vi "Determine Controller.vi"(7 "Processing In":refnum<class "Processing.lvclass">, 11 "PathRegex Router in":refnum<class "PathRegex Router.lvclass">) -> (0 "error out":errorcluster, 2 "Controller":refnum<class "Controller.lvclass">, 5 "Processing":refnum<class "Processing.lvclass">)   [LabVIEW 2020, in "HTTP Server.lvlib" / "PathRegex Router.lvclass"]
uses:
  PathRegex Router.lvclass
  PathRegex Router.lvclass/PathRegex Router.ctl
  lv-http-util/HTTP Utils/Request/Request.lvclass
  Controller/Controller.lvclass
  Processing/Processing.lvclass
  lv-uri/URI/URI/URI.lvclass
  lv-uri/URI/URI.lvlib
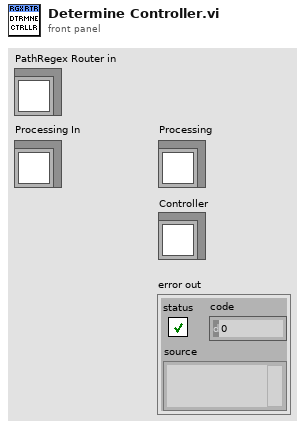
[diagram p1: front panel]
types:
  T1 = typedef "HTTP Server.lvlib/Controller Map.ctl" = map{T2, refnum<class "Controller.lvclass">}
  T2 = typedef "HTTP Server.lvlib/Priority.ctl" = cluster{"Entity":u16, "Index":u16}
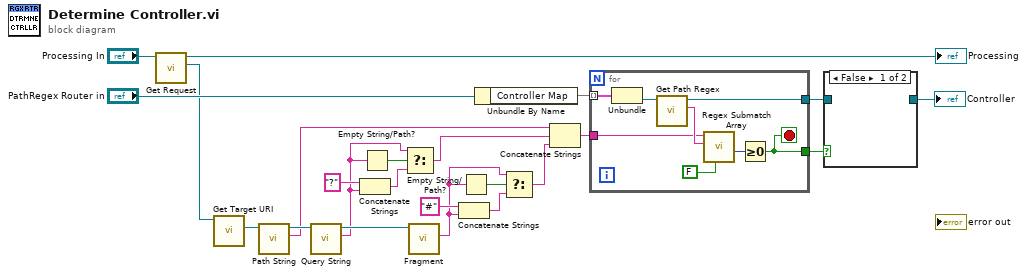
[diagram p0: block diagram]
diagram:
  n1 = call "Get Request.vi"("Processing in"="Processing In") -> ("Request"=w3:refnum<class "Request.lvclass">, "Processing out"=→"Processing":refnum<class "Processing.lvclass">)  [unwired: 9 in]
  n2 = call "Get Target URI.vi"("Request in"=w3) -> ("Target URI"=w22:refnum<class "URI.lvclass">)  [unwired: 8 in, 2 out]
  n3 = call "Path String.vi"("URI in"=w22) -> ("Path String"=w19:string, "URI out"=w21:refnum<class "URI.lvclass">)  [unwired: 9 in]
  n4 = call "Query String.vi"("URI in"=w21) -> ("Query String"=w7:string, "URI out"=w20:refnum<class "URI.lvclass">)  [unwired: 9 in]
  n5 = Concatenate Strings("?" ("string"), w7) -> (w8:string)
  n6 = Empty String/Path?(string/path=w7) -> (empty?=w9:bool)
  n7 = Select(t=w7, s=w9, f=w8) -> (s? t:f=w6:string)
  n8 = call "Fragment.vi"("URI in"=w20) -> ("Fragment"=w11:string)  [unwired: 9 in, 1 out]
  n9 = Concatenate Strings("#" ("string"), w11) -> (w12:string)
  n10 = Empty String/Path?(string/path=w11) -> (empty?=w14:bool)
  n11 = Unbundle By Name("PathRegex Router in") -> ("Controller Map"=w17:T1)
  n12 = Select(t=w11, s=w14, f=w12) -> (s? t:f=w5:string)
  n13 = Concatenate Strings(w19, w6, w5) -> (w18:string)
  n14 = for {
    tunnel: w18 -> [w28]
    tunnel: w17 -> [w31] mode=indexing
    tunnel: [w25] -> w16
    tunnel: [w24] -> w15
    stop <- w25 stop-if-true
    n15 = Unbundle(w31) -> ("Controller"=w30:refnum<class "Controller.lvclass">)  [unwired: 1 out]
    n16 = call-dynamic "Get Path Regex.vi"("Controller in"=w30) -> ("Path Regex"=w29:string, "Controller out"=w24:refnum<class "Controller.lvclass">)  [unwired: 8 in, 1 out]
    n17 = call "Regex Submatch Array.vi"("Submatches? (T)"=FALSE, "regular expression"=w29, "string"=w28) -> ("offset past match"=w26:i32)  [unwired: 4 in, 4 out]
    n18 = Greater Or Equal To 0?(x=w26) -> (x >= 0?=w25:bool)
  }
  n19 = case shown="False" w16 {
    tunnel: w15 -> [_ w32]
    tunnel: [_ w32] -> w1
    frame False {
    }
    frame True {
    }
  }
  "Controller" <- w1
